vi "Calculate Pump Power.vi"(1 "Motor temperature 2":u8, 2 "Motor temperature":u8, 3 "Acceleration pedal":dbl) -> (0 "Pumps power":dbl(slide) scale=0.0..100.0 scale format="%#_g%%")   [LabVIEW 2016]
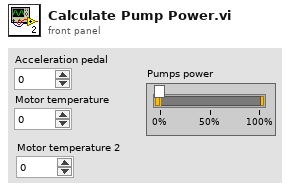
[diagram p1: front panel]
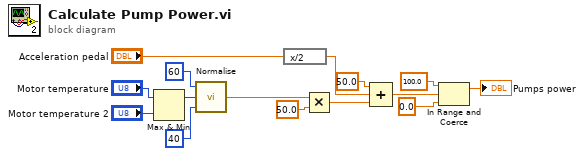
[diagram p0: block diagram]
diagram:
  n1 = Max & Min(x="Motor temperature", y="Motor temperature 2") -> (max(x,y)=w8:u8)  [unwired: 1 out]
  n2 = call "Normalise.vi"("min"=u8 40 ("lower limit"), "value"=w8, "max"=u8 60 ("upper limit")) -> ("normalised"=w7:dbl)  [unwired: 2 out]
  n3 = expression code="x/2"("Acceleration pedal") -> (w15:dbl)
  n4 = Multiply(x=w7, y=50.0) -> (x*y=w5:dbl)
  n5 = Compound Arithmetic op=ADD(50.0 ("value"), w15, w5) -> (w4:dbl)
  n6 = In Range and Coerce(upper limit=100.0, x=w4, lower limit=0.0) -> (coerced(x)=→"Pumps power":dbl)  [unwired: 1 out]
